vi "FTW-CodeGen-AdaptToInputs.vi"(0 "State In":T1 {"Actor Interface"."Bounds"."Left" format="%dpx"; "Actor Interface"."Bounds"."Top" format="%dpx"; "Actor Interface"."Bounds"."Right" format="%dpx"; "Actor Interface"."Bounds"."Bottom" format="%dpx"}, 5 "XRef":refnum<vi>, 7 "Term Types":cluster{"Type":variant, "ID":string}[](array[cluster])) -> (4 "State Out":T1 {"Actor Interface"."Bounds"."Left" format="%dpx"; "Actor Interface"."Bounds"."Top" format="%dpx"; "Actor Interface"."Bounds"."Right" format="%dpx"; "Actor Interface"."Bounds"."Bottom" format="%dpx"}, 6 "Reply":string[](array[string]))   [LabVIEW 2014, in "FTW-Actor-Spawn.xnode"]
uses:
  FTW-Actor-Spawn.xnode
  FTW-CodeGen-State.ctl
  FTW-CodeGen-XNodeReplyType.ctl
  src/reflection/FTW-Reflection-Types.ctl
panel:
  # "Inputs"
  # "Outputs"
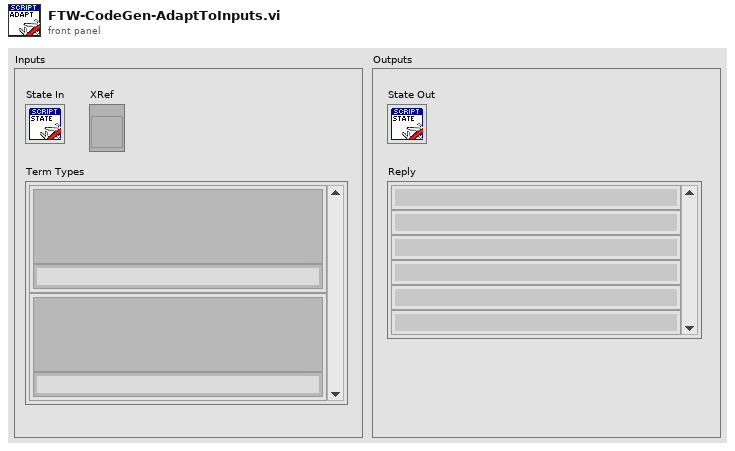
[diagram p1: front panel]
types:
  T1 = typedef "FTW-Actor-Spawn.xnode/FTW-CodeGen-State.ctl" = cluster{"Path Wired?":bool, "Actor Interface":cluster{"Name":string, "Type":variant, "Bounds":cluster{"Left":i32, "Top":i32, "Right":i32, "Bottom":i32}, "Input":bool, "Recommended":bool, "Required":bool, "Dynamic Dispatch":bool, "On Interface":bool, "\"The\" Config Terminal":bool}[], "Config Terminal Index":i32}
  T2 = typedef "FTW-CodeGen-XNodeReplyType.ctl" = enum16{"UpdateState", "AdaptToInputs", "AdaptAndAugment", "CosmeticUpdate", "NoReply"}
  T3 = cluster{"Name":string, "Type":variant, "Bounds":cluster{"Left":i32, "Top":i32, "Right":i32, "Bottom":i32}, "Input":bool, "Recommended":bool, "Required":bool, "Dynamic Dispatch":bool, "On Interface":bool, "\"The\" Config Terminal":bool}[]
  T4 = cluster{"Name":string, "Type":variant, "Bounds":cluster{"Left":i32, "Top":i32, "Right":i32, "Bottom":i32}, "Input":bool, "Recommended":bool, "Required":bool, "Dynamic Dispatch":bool, "On Interface":bool, "\"The\" Config Terminal":bool}
  T5 = typedef "FTW-Reflection-ConPaneInterface-Terminal.ctl" = cluster{"Name":string, "LabVIEW Type":T6, "Datatype":variant, "Bounds":cluster{"Left":i32, "Top":i32, "Right":i32, "Bottom":i32}, "Input Stomp Index":i32, "Input":bool, "Wired":bool, "Dynamic Dispatch":bool, "Recommended":bool, "Required":bool, "Stomped":bool, "RSV20":bool, "RSV40":bool}
  T6 = typedef "FTW-Reflection-Types.ctl" = enum16{"Unknown", "Void", "Array", "Cluster", "LVObject", "Boolean", "I8", "I16", "I32", "I64", "U8", "U16", "U32", "U64", "SGL", "DBL", "EXT", "CSG", "CDB", "CXT", "FXP", "EnumU8", "EnumU16", "EnumU32", "EnumU64", "SGLwithUnit", "DBLwithUnit", "EXTwithUnit", "CSGwithUnit", "CDBwithUnit", "CXTwithUnit", "String", "Path", "Picture", "Tag", "LVVariant", "Timestamp", "WaveformI8", "WaveformI16", "WaveformI32", "WaveformI64", "WaveformU8", "WaveformU16", "WaveformU32", "WaveformU64", "WaveformSGL", "WaveformDBL", "WaveformEXT", "WaveformCSG", "WaveformCDB", "WaveformCXT", "WaveformDigital", "WaveformUnknownType", "DigitalData", "DynamicData", "ExternalData", "FileByteStream", "TDMStream", "dotNET", "ActiveX", "VIServerReference", "VIReference", "ApplicationInstance", "Menu", "ConnectionDataSocket", "ConnectionVISA", "ConnectionBluetooth", "ConnectionIrDA", "ConnectionTCP", "ConnectionUDP", "ConnectionHTTPClient", "ConnectionFTP", "Occurrence", "Notifier", "Queue", "Rendezvous", "Semaphore", "RTFIFO", "EventPublisher", "EventRegistration", "EventCallback", "DataValueReference", "GenericClass", "GenericClassTag", "GenericClassDeepCopy", "GenericClassFlattened", "GenericClassTagFlattened", "GenericReferenceType", "WindowsRegistry", "OverloadedDatalogRef", "ReferenceUnknownType", "ByteArray", "ConPaneInterface"}
  T7 = cluster{"Left":i32, "Top":i32, "Right":i32, "Bottom":i32}
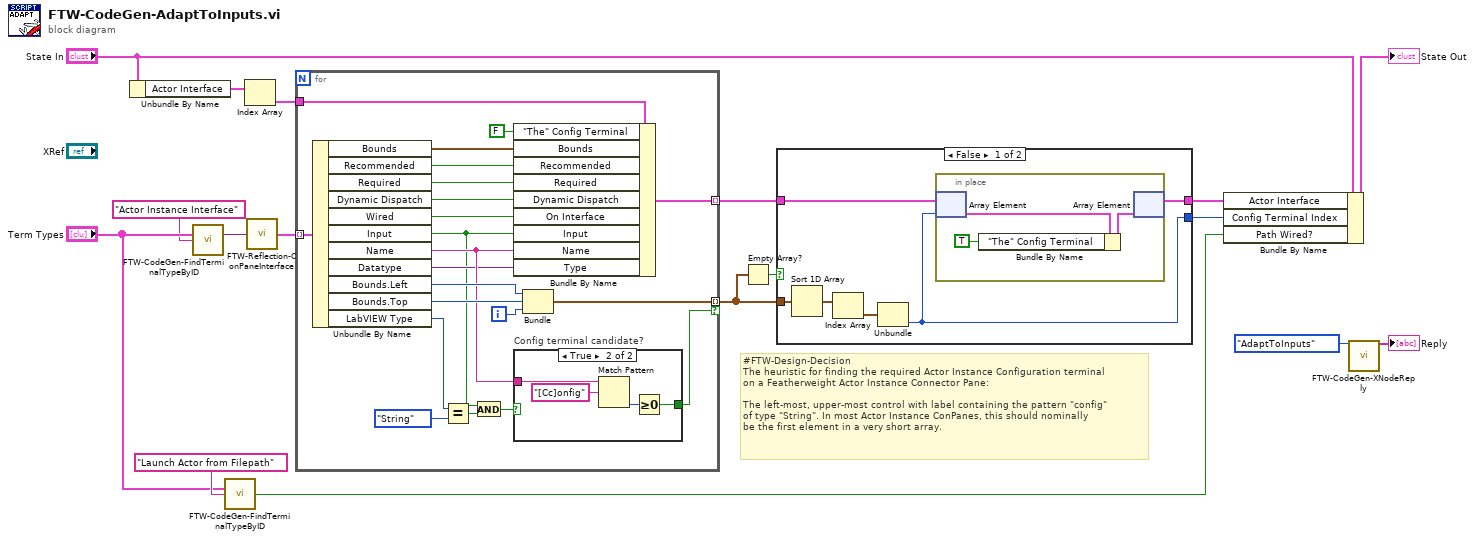
[diagram p0: block diagram]
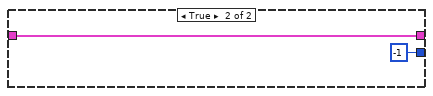
[diagram p2: hidden frame]
diagram:
  # "#FTW-Design-Decision\nThe heuristic for finding the required Actor Instance Configuration terminal\non a Featherweight Actor Instance Connector Pane:\n\nThe left-most, upper-most control with label containing the pattern \"config\"\nof type \"String\". In most Actor Instance ConPanes, this should nominally\nbe the first element in a very short array."
  n1 = Unbundle By Name("State In") -> ("Actor Interface"=w9:T3)
  n2 = call "FTW-CodeGen-FindTerminalTypeByID.vi"("Terminals"="Term Types", "Terminal ID"="Actor Instance Interface") -> ("Terminal Type"=w11:variant)  [unwired: 12 in, 1 out]
  n3 = call "FTW-CodeGen-FindTerminalTypeByID.vi"("Terminals"="Term Types", "Terminal ID"="Launch Actor from Filepath") -> ("Found?"=w6:bool)  [unwired: 12 in, 1 out]
  n4 = Index Array(array=w9) -> (element=w8:T4)  [unwired: 1 in]
  n5 = call "FTW-Reflection-ConPaneInterface.vi"("VI Connector Pane (or VI Reference)"=w11) -> ("Terminals"=w7:T5[])  [unwired: 12 in, 2 out]
  n6 = for {
    tunnel: w8 -> [w38]
    tunnel: [w37] -> w2 mode=indexing
    tunnel: w7 -> [w36] mode=indexing
    tunnel: [w27] -> w5 mode=indexing if=w26
    i -> [w28]
    n7 = Unbundle By Name(w36) -> ("Bounds"=w35:T7, "Recommended"=w34:bool, "Required"=w33:bool, "Dynamic Dispatch"=w32:bool, "Wired"=w31:bool, "Input"=w19:bool, "Name"=w24:string, "Datatype"=w23:variant, "Bounds.Left"=w30:i32, "Bounds.Top"=w29:i32, "LabVIEW Type"=w22:T6)
    n8 = Equal?(x=w22, y=FTW-Reflection-Types."String") -> (x = y?=w20:bool)
    n9 = And(x=w19, y=w20) -> (x .and. y?=w18:bool)
    n10 = Bundle By Name(cluster=w38, "\"The\" Config Terminal"=FALSE ("\"The\" Config Terminal"), "Bounds"=w35, "Recommended"=w34, "Required"=w33, "Dynamic Dispatch"=w32, "On Interface"=w31, "Input"=w19, "Name"=w24, "Type"=w23) -> (w37:T4)
    n11 = case "Config terminal candidate?" shown="True" w18 {
      tunnel: w24 -> [_ w42]
      tunnel: [_ w41] -> w26
      frame False {
      }
      frame True {
        n12 = Match Pattern(string=w42, regular expression="[Cc]onfig") -> (offset past match=w39:i32)  [unwired: 1 in, 3 out]
        n13 = Greater Or Equal To 0?(x=w39) -> (x >= 0?=w41:bool)
      }
    }
    n14 = Bundle("Left"=w30, "Top"=w29, w28) -> (w27:cluster{"Left":i32, "Top":i32, i32})  [unwired: 1 in]
  }
  n15 = Empty Array?(array=w5) -> (empty?=w4:bool)
  n16 = case shown="False" w4 {
    tunnel: w5 -> [w46 _]
    tunnel: [w44 w53] -> w3
    tunnel: w2 -> [w45 w53]
    tunnel: [w43 -1] -> w1
    frame False {
      n17 = Sort 1D Array(array=w46) -> (sorted array=w48:cluster{"Left":i32, "Top":i32, i32}[])
      n18 = Index Array(array=w48) -> (element=w47:cluster{"Left":i32, "Top":i32, i32})  [unwired: 1 in]
      n19 = Unbundle(w47) -> (w43:i32)  [unwired: 2 out]
      n20 = in-place {
        n21 = in-place-array #1(w45, w43) -> (w51:T4)
        n22 = Bundle By Name(cluster=w51, "\"The\" Config Terminal"=TRUE ("\"The\" Config Terminal")) -> (w50:T4)
        n23 = in-place-array #1(w50) -> (w44:T3)  [unwired: 1 out]
      }
    }
    frame True {
    }
  }
  n24 = Bundle By Name(cluster="State In", "Actor Interface"=w3, "Config Terminal Index"=w1, "Path Wired?"=w6) -> (→"State Out":T1)
  n25 = call "FTW-CodeGen-XNodeReply.vi"("XNode Reply Type"=FTW-CodeGen-XNodeReplyType."AdaptToInputs") -> ("Reply"=→"Reply":string[])  [unwired: 14 in]
